vi "MonitorThreshold.vi"(8 "error constant":errorcluster, 9 "CalcData":T7, 10 "CaliData":T8 caption="All Data Cluster", 11 "Data":T1={"State"=enum."APU Select", "2D User Info"=[], "APU Setup File"={"Sensor Info"=[], "Variables"=[], "CMM Table 106"=[], "CMM Table 106B "=[], "Accel Config"=[], "Report Sheet 1"=[], "Report Sheet 2"=[], "Report Sheet 3"=[]}, "Test Information"={"APU Part Number:"="", "Model:"="", "Serial Number:"="", "Customer:"="", "Work Order:"="", "Pre or Post SB"="", "Run Count"=0, "APU Selected"="<Select>"}, "ChannelTags"=[], "Live_Min_Max_Dev"=[], "CalChannels"=[], "Slopes"=[], "Offsets"=[], "Calculated Values"={"C.00"=0.0, "C.01"=0.0, "C.02"=0.0, "C.03"=0.0, "C.04"=0.0, "C.05"=0.0, "C.06"=0.0, "C.07"=0.0, "C.08"=0.0, "C.09"=0.0, "C.10"=0.0, "C.11"=0.0, "C.12"=0.0, "C.13"=0.0, "C.14"=0.0, "C.15"=0.0, "C.16"=0.0, "C.17"=0.0, "C.18"=0.0, "C.19"=0.0, "C.20"=0.0, "C.21"=0.0, "C.22"=0.0, "C.23"=0.0, "C.24"=0.0, "C.25"=0.0, "C.26"=0.0, "C.27"=0.0, "C.28"=0.0, "C.29"=0.0, "C.30"=0.0, "C.31"=0.0, "C.32"=0.0, "C.33"=0.0, "C.34"=0.0, "C.35"=0.0, "C.36"=0.0, "C.37"=0.0, "C.38"=0.0, "C.39"=0.0, "C.40"=0.0, "C.41"=0.0, "C.42"=0.0, "C.43"=0.0, "C.44"=0.0, "C.45"=0.0, "C.46"=0.0, "C.47"=0.0, "C.48"=0.0, "C.49"=0.0, "C.50"=0.0, "C.51"=0.0, "C.52"=0.0, "C.53"=0.0, "C.54"=0.0, "C.55"=0.0, "C.56"=0.0, "C.57"=0.0, "C.58"=0.0, "C.59"=0.0, "C.60"=0.0, "C.61"=0.0, "C.62"=0.0}, "ThresholdChannels"=[], "ThresholdRPM"=[], "ThresholdMin"=[], "ThresholdValue"=[], "HeavyCCM"=[], "LightCCM"=[], "FuelFarm"=FALSE} {"Test Information"."Run Count" min=0 step=1}) -> (0 "error out":errorcluster)   [LabVIEW 2018, in "Controller (Host).lvlib"]
uses:
  Controller (Host).lvlib
  Top Level/Shared Controls/All Data Cluster.ctl
  Top Level/Shared Controls/Acq Data.ctl
  Top Level/Shared Controls/Calculated Data.ctl
  Private Controls/Controller (Host) Data.ctl
  Private Controls/State.ctl
  Top Level/Shared Controls/APU Setup File.ctl
  Public Controls/Test Information.ctl
  Public VIs/PreorPostSB.ctl
  Public Controls/APU Select.ctl
  Testing UI 1/Testing UI 1.lvlib
panel:
  out "Error Out":errorcluster
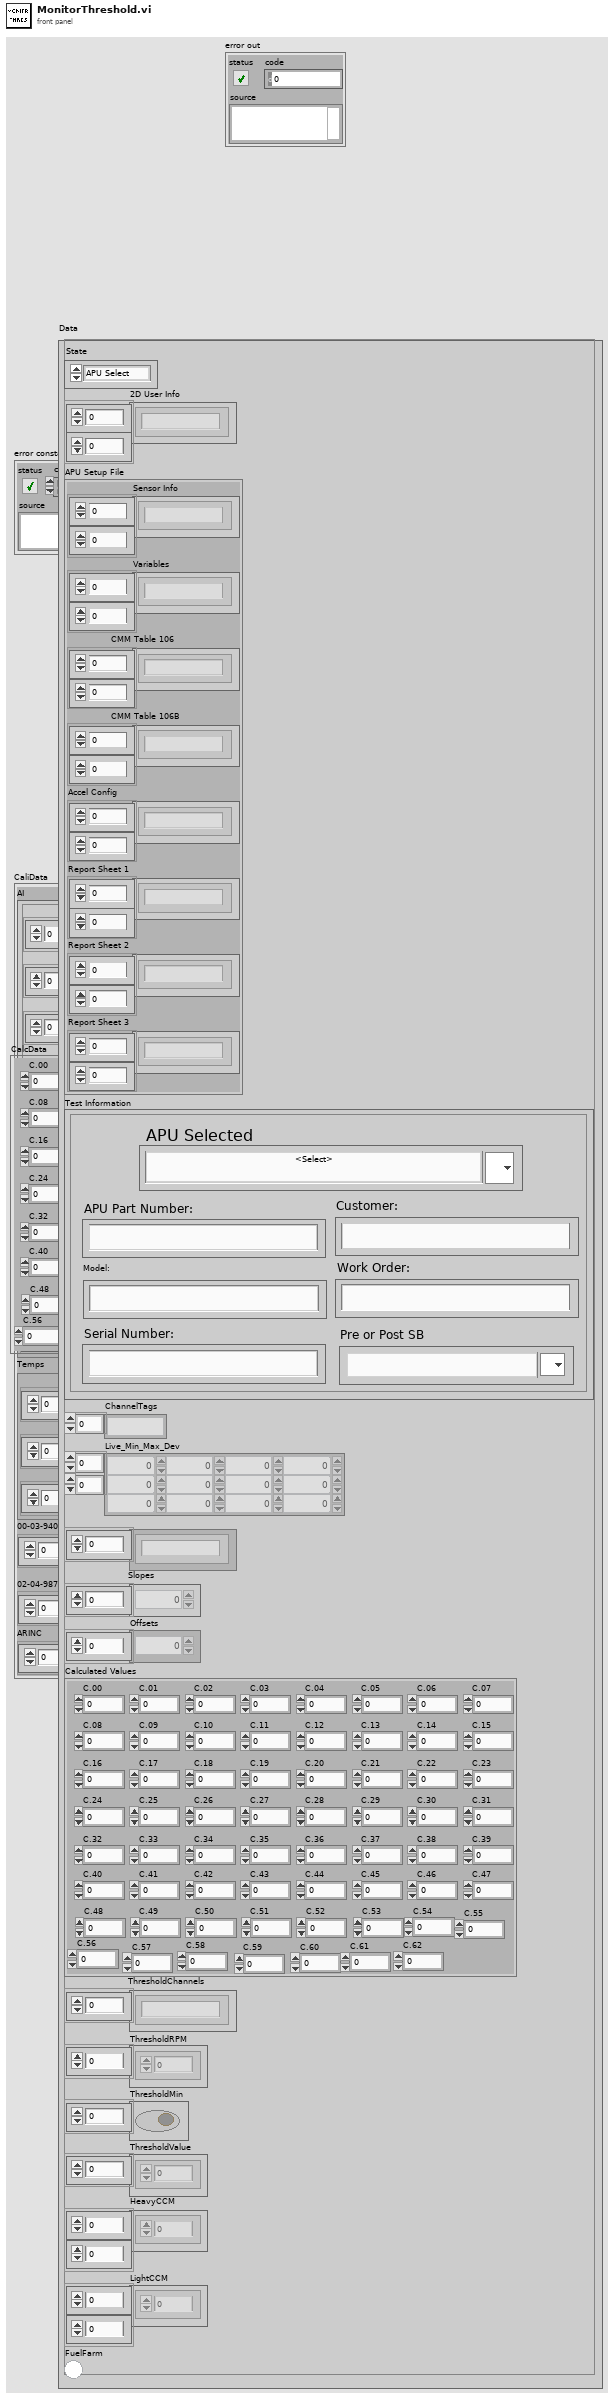
[diagram p1: front panel]
types:
  T1 = typedef "Controller (Host).lvlib/Controller (Host) Data.ctl" = cluster{"State":T2, "2D User Info":string[][], "APU Setup File":T3, "Test Information":T4, "ChannelTags":string[], "Live_Min_Max_Dev":dbl[][], "CalChannels":string[], "Slopes":dbl[], "Offsets":dbl[], "Calculated Values":T7, "ThresholdChannels":string[], "ThresholdRPM":dbl[], "ThresholdMin":bool[], "ThresholdValue":dbl[], "HeavyCCM":dbl[][], "LightCCM":dbl[][], "FuelFarm":bool}
  T2 = typedef "Controller (Host).lvlib/State.ctl" = enum16{"APU Select", "Operation Select", "SubTests Select", "Calibration", "Testing", "Exit"}
  T3 = typedef "APU Setup File.ctl" = cluster{"Sensor Info":string[][], "Variables":string[][], "CMM Table 106":string[][], "CMM Table 106B ":string[][], "Accel Config":string[][], "Report Sheet 1":string[][], "Report Sheet 2":string[][], "Report Sheet 3":string[][]}
  T4 = typedef "Controller (Host).lvlib/Test Information.ctl" = cluster{"APU Part Number:":string, "Model:":string, "Serial Number:":string, "Customer:":string, "Work Order:":string, "Pre or Post SB":T5, "Run Count":i32, "APU Selected":T6}
  T5 = typedef "Controller (Host).lvlib/PreorPostSB.ctl" = string
  T6 = typedef "Controller (Host).lvlib/APU Select.ctl" = string
  T7 = typedef "Calculated Data.ctl" = cluster{"C.00":dbl, "C.01":dbl, "C.02":dbl, "C.03":dbl, "C.04":dbl, "C.05":dbl, "C.06":dbl, "C.07":dbl, "C.08":dbl, "C.09":dbl, "C.10":dbl, "C.11":dbl, "C.12":dbl, "C.13":dbl, "C.14":dbl, "C.15":dbl, "C.16":dbl, "C.17":dbl, "C.18":dbl, "C.19":dbl, "C.20":dbl, "C.21":dbl, "C.22":dbl, "C.23":dbl, "C.24":dbl, "C.25":dbl, "C.26":dbl, "C.27":dbl, "C.28":dbl, "C.29":dbl, "C.30":dbl, "C.31":dbl, "C.32":dbl, "C.33":dbl, "C.34":dbl, "C.35":dbl, "C.36":dbl, "C.37":dbl, "C.38":dbl, "C.39":dbl, "C.40":dbl, "C.41":dbl, "C.42":dbl, "C.43":dbl, "C.44":dbl, "C.45":dbl, "C.46":dbl, "C.47":dbl, "C.48":dbl, "C.49":dbl, "C.50":dbl, "C.51":dbl, "C.52":dbl, "C.53":dbl, "C.54":dbl, "C.55":dbl, "C.56":dbl, "C.57":dbl, "C.58":dbl, "C.59":dbl, "C.60":dbl, "C.61":dbl, "C.62":dbl}
  T8 = typedef "All Data Cluster.ctl" = cluster{"AI":T9, "Accel Data":cluster{"Accel RMS(in/sec2)":dbl[], "Accel Peak(in/sec2)":dbl[], "Velocity RMS(in/sec)":dbl[], "Velocity Peak(in/sec)":dbl[]}, "Temps":cluster{"01-00-9213":dbl[], "01-01-9213":dbl[], "01-02-9213":dbl[]}, "00-03-9402(RPM)":dbl[], "02-04-9871":dbl[], "ARINC":sgl[]}
  T9 = typedef "Acq Data.ctl" = cluster{"00-00-9220":dbl[], "00-01-9220":dbl[], "02-02-9219":dbl[], "02-03-9227":dbl[], "02-05-9205":dbl[]}
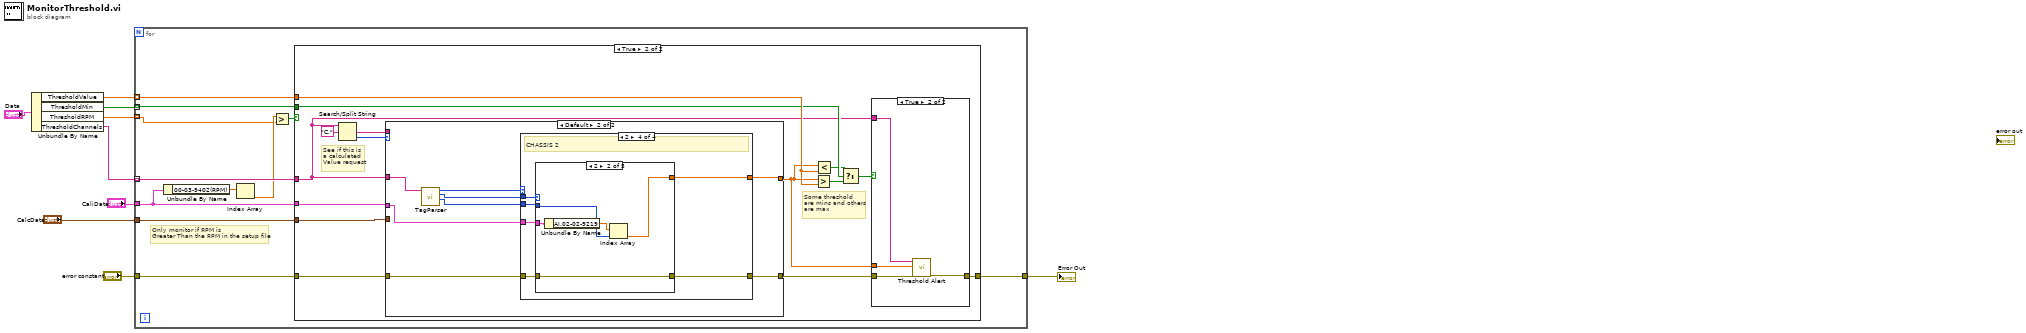
[diagram p0: block diagram]
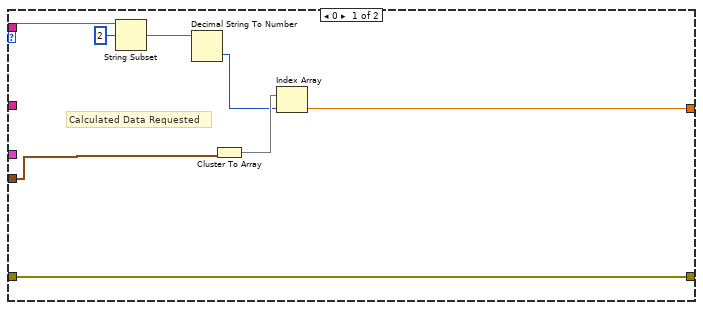
[diagram p4: hidden frame]
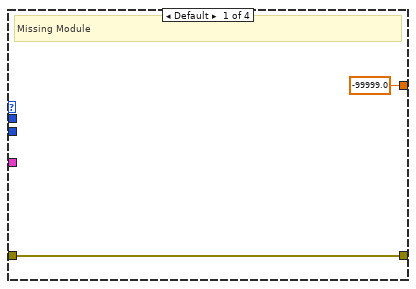
[diagram p5: hidden frame]
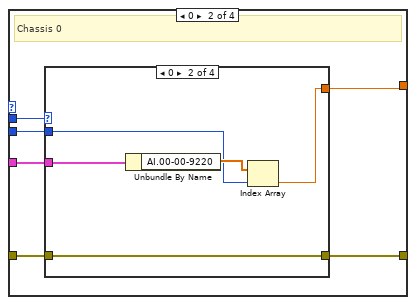
[diagram p6: hidden frame]
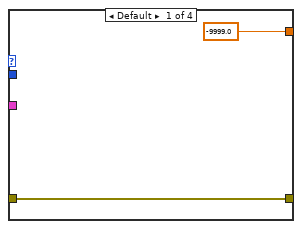
[diagram p7: hidden frame]
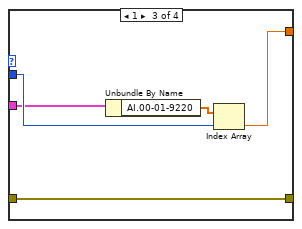
[diagram p8: hidden frame]
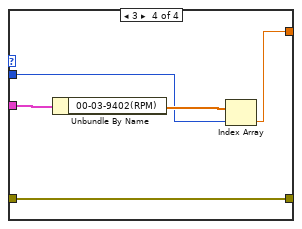
[diagram p9: hidden frame]
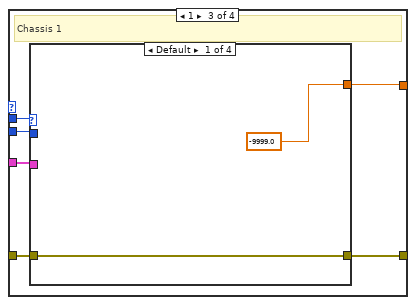
[diagram p10: hidden frame]
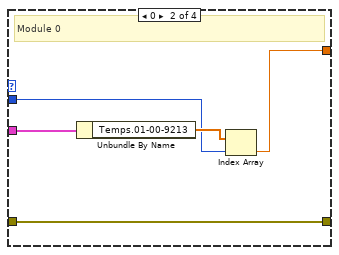
[diagram p11: hidden frame]
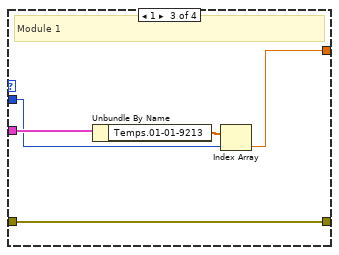
[diagram p12: hidden frame]
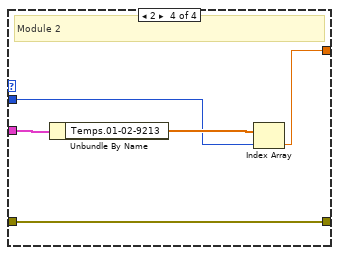
[diagram p13: hidden frame]
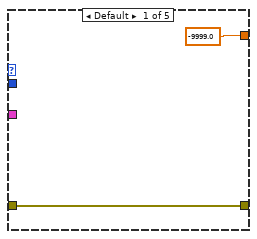
[diagram p14: hidden frame]
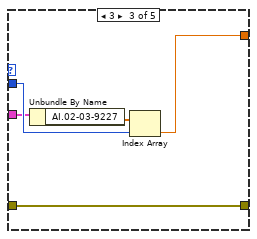
[diagram p15: hidden frame]
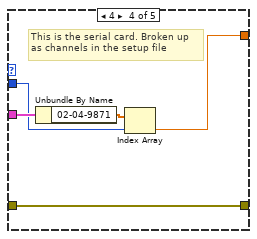
[diagram p16: hidden frame]
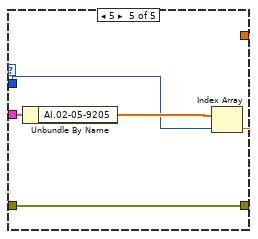
[diagram p17: hidden frame]
diagram:
  n1 = Unbundle By Name("Data") -> ("ThresholdValue"=w3:dbl[], "ThresholdMin"=w2:bool[], "ThresholdRPM"=w1:dbl[], "ThresholdChannels"=w4:string[])
  n2 = for {
    tunnel: w4 -> [w19] mode=indexing
    tunnel: "error constant" -> [w20]
    tunnel: [w18] -> w9
    tunnel: "CaliData" -> [w16]
    tunnel: "CalcData" -> [w17]
    tunnel: w3 -> [w13] mode=indexing
    tunnel: w2 -> [w12] mode=indexing
    tunnel: w1 -> [w10] mode=indexing
    # "Only monitor if RPM is \nGreater Than the RPM in the setup file"
    n3 = Unbundle By Name(w16) -> ("00-03-9402(RPM)"=w15:dbl[])
    n4 = Index Array(array=w15) -> (element=w11:dbl)  [unwired: 1 in]
    n5 = Greater?(x=w11, y=w10) -> (0:w14:bool)
    n6 = case shown="True" w14 {
      tunnel: w20 -> [w21 w36]
      tunnel: w19 -> [_ w23]
      tunnel: [w21 w26] -> w18
      tunnel: w17 -> [_ w32]
      tunnel: w16 -> [_ w31]
      tunnel: w13 -> [_ w30]
      tunnel: w12 -> [_ w29]
      frame False {
      }
      frame True {
        # "Some threshold\nare mins and others\nare max"
        # "See if this is\na calculated\nValue request"
        n7 = Search/Split String(string=w23, search string/char (-)="C.") -> (match + rest of string=w33:string, offset of match=w34:i32)  [unwired: 1 in, 1 out]
        n8 = case shown="Default" w34 {
          tunnel: w23 -> [_ w53]
          tunnel: w33 -> [w49 _]
          tunnel: w31 -> [_ w57]
          tunnel: w36 -> [w44 w56]
          tunnel: [w44 w55] -> w25
          tunnel: w32 -> [w43 _]
          tunnel: [w42 w54] -> w22
          frame 0 {
            # "Calculated Data Requested"
            n9 = String Subset(string=w49, offset (0)=2) -> (substring=w47:string)  [unwired: 1 in]
            n10 = Decimal String To Number(string=w47) -> (number=w45:i32)  [unwired: 2 in, 1 out]
            n11 = Cluster To Array(cluster=w43) -> (array=w46:dbl[])
            n12 = Index Array(array=w46, index=w45) -> (element=w42:dbl)
          }
          frame Default {
            n13 = call "TagParser.vi"("Channel Tag"=w53) -> ("Channel"=w50:i32, "Module"=w51:i32, "Chassis"=w52:i32)  [unwired: 8 in]
            n14 = case shown="2" w52 {
              tunnel: w51 -> [_ w65 w86 w110]
              tunnel: w57 -> [_ w64 w88 w109]
              tunnel: w50 -> [_ w63 w87 w111]
              tunnel: w56 -> [w58 w62 w84 w108]
              tunnel: [w58 w61 w85 w107] -> w55
              tunnel: [-99999.0 ("Numeric") w60 w83 w106] -> w54
              frame Default {
                # "Missing Module"
              }
              frame 0 {
                # "Chassis 0"
                n15 = case shown="0" w65 {
                  tunnel: w64 -> [_ w68 w73 w82]
                  tunnel: w63 -> [_ w71 w76 w80]
                  tunnel: [-9999.0 ("Numeric") w70 w75 w79] -> w60
                  tunnel: w62 -> [w66 w69 w74 w78]
                  tunnel: [w66 w69 w74 w78] -> w61
                  frame Default {
                  }
                  frame 0 {
                    n16 = Unbundle By Name(w68) -> ("AI.00-00-9220"=w72:dbl[])
                    n17 = Index Array(array=w72, index=w71) -> (element=w70:dbl)
                  }
                  frame 1 {
                    n18 = Unbundle By Name(w73) -> ("AI.00-01-9220"=w77:dbl[])
                    n19 = Index Array(array=w77, index=w76) -> (element=w75:dbl)
                  }
                  frame 3 {
                    n20 = Unbundle By Name(w82) -> ("00-03-9402(RPM)"=w81:dbl[])
                    n21 = Index Array(array=w81, index=w80) -> (element=w79:dbl)
                  }
                }
              }
              frame 1 {
                # "Chassis 1"
                n22 = case shown="Default" w86 {
                  tunnel: w88 -> [_ w95 w100 w105]
                  tunnel: w87 -> [_ w93 w98 w103]
                  tunnel: [-9999.0 ("Numeric") w92 w97 w102] -> w83
                  tunnel: [w89 w91 w96 w101] -> w85
                  tunnel: w84 -> [w89 w91 w96 w101]
                  frame Default {
                  }
                  frame 0 {
                    # "Module 0"
                    n23 = Unbundle By Name(w95) -> ("Temps.01-00-9213"=w94:dbl[])
                    n24 = Index Array(array=w94, index=w93) -> (element=w92:dbl)
                  }
                  frame 1 {
                    # "Module 1"
                    n25 = Unbundle By Name(w100) -> ("Temps.01-01-9213"=w99:dbl[])
                    n26 = Index Array(array=w99, index=w98) -> (element=w97:dbl)
                  }
                  frame 2 {
                    # "Module 2"
                    n27 = Unbundle By Name(w105) -> ("Temps.01-02-9213"=w104:dbl[])
                    n28 = Index Array(array=w104, index=w103) -> (element=w102:dbl)
                  }
                }
              }
              frame 2 {
                # "CHASSIS 2"
                n29 = case shown="2" w110 {
                  tunnel: w109 -> [_ w118 w119 w128 w129]
                  tunnel: w111 -> [_ w116 w122 w126 w132]
                  tunnel: [-9999.0 ("Numeric") w115 w121 w125 w131] -> w106
                  tunnel: w108 -> [w112 w114 w120 w124 w130]
                  tunnel: [w112 w114 w120 w124 w130] -> w107
                  frame Default {
                  }
                  frame 2 {
                    n30 = Unbundle By Name(w118) -> ("AI.02-02-9219"=w117:dbl[])
                    n31 = Index Array(array=w117, index=w116) -> (element=w115:dbl)
                  }
                  frame 3 {
                    n32 = Unbundle By Name(w119) -> ("AI.02-03-9227"=w123:dbl[])
                    n33 = Index Array(array=w123, index=w122) -> (element=w121:dbl)
                  }
                  frame 4 {
                    # "This is the serial card. Broken up \nas channels in the setup file"
                    n34 = Unbundle By Name(w128) -> ("02-04-9871"=w127:dbl[])
                    n35 = Index Array(array=w127, index=w126) -> (element=w125:dbl)
                  }
                  frame 5 {
                    n36 = Unbundle By Name(w129) -> ("AI.02-05-9205"=w133:dbl[])
                    n37 = Index Array(array=w133, index=w132) -> (element=w131:dbl)
                  }
                }
              }
            }
          }
        }
        n38 = Greater?(x=w22, y=w30) -> (0:w27:bool)
        n39 = Less?(x=w22, y=w30) -> (x < y?=w28:bool)
        n40 = Select(t=w28, s=w29, f=w27) -> (s? t:f=w24:bool)
        n41 = case shown="True" w24 {
          tunnel: [w37 w40] -> w26
          tunnel: w25 -> [w37 w41]
          tunnel: w23 -> [_ w38]
          tunnel: w22 -> [_ w39]
          frame False {
            # "All Good"
          }
          frame True {
            n42 = call "Threshold Alert.vi"("error in (no error)"=w41, "Value"=w39, "Message"=w38) -> ("error out"=w40:errorcluster)  [unwired: 8 in]
          }
        }
      }
    }
  }
  "Error Out" <- w9
